vi "Update Indicator Value.vi"(8 "error in (no error)":errorcluster, 9 "uService Template in":refnum<class "Father of all uServices.lvclass">, 10 "Item data":variant, 11 "Control in":refnum<vi>) -> (0 "error out":errorcluster, 3 "Control out":refnum<vi>)   [LabVIEW 2026, in "TALOS.lvlib" / "Father of all uServices.lvlib" / "Father of all uServices.lvclass"]
uses:
  Father of all uServices.lvclass
  Ancestor/Ancestor/Ancestor.lvclass/Ancestor.ctl
  Support VIs/Generate Error.vi
  FGV/Error Memory/Get Error Description.vi
  Support VIs/Get PC name.vi
  Ancestor/Ancestor/Read ID.vi
  Support VIs/Get Class Name.vi
  FGV/Error Memory/Error Memory Core.vi
  <vilib>/AdvancedString/Delimited String to 1D String Array.vi
  <vilib>/AdvancedString/Delimited String to 1D String Array (string).vi
  Support VIs/Circus Root Path.vi
  FGV/Error Memory/Error Crt Lvl checker.vi
  FGV/Error Memory/Error Memory Core.vi/40c8088d-b597-4017-91af-faa98e00292e.vi
  FGV/Error Memory/Error Memory Core.vi/d4a3ab98-063c-4e44-b43d-fbdcfe6c2be2.vi
  Support VIs/Global Memory.vi
  <vilib>/Utility/LVClass/Get LV Class Name.vi
  Support VIs/Is in Packed Library.vi
  Support VIs/TALOS Root path.vi
  Support VIs/Read CSV worksheet.vi
  Support VIs/Global Constants.vi
  <vilib>/Utility/error.llb/General Error Handler.vi
  Support VIs/Error Log.vi
  Ancestor/Ancestor/Ancestor.lvclass
  <vilib>/Comparison/Equal/Equal Functor/Equal Functor.lvclass
  TALOS.lvlib
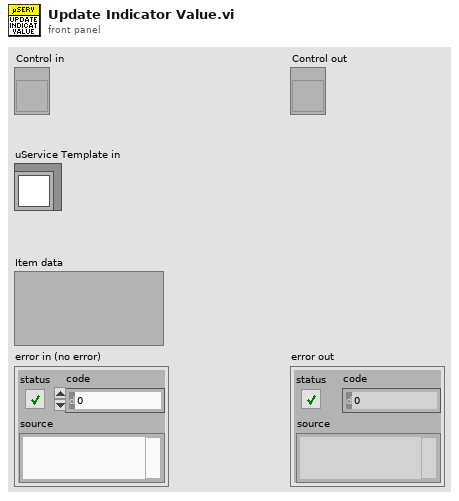
[diagram p1: front panel]
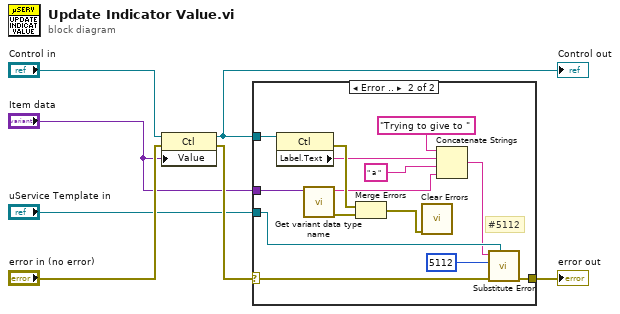
[diagram p0: block diagram]
diagram:
  n1 = property class="Ctl"(reference="Control in", error in="error in (no error)", "Value"="Item data") -> (reference out=w3:refnum<vi>, error out=w5:errorcluster)
  "Control out" <- w3
  n2 = case shown="Error .." w5 {
    selector: w5 -> [w8 w22]
    tunnel: [w8 w21] -> w4
    tunnel: w3 -> [_ w20]
    tunnel: "uService Template in" -> [_ w18]
    tunnel: "Item data" -> [_ w17]
    frame No Error {
    }
    frame Error {
      # "#5112"
      n3 = property class="Ctl"(reference=w20) -> (error out=w16:errorcluster, "Label.Text"=w12:string)  [unwired: 1 in, 1 out]
      n4 = call "Get variant data type name.vi"("variant"=w17) -> ("error out"=w15:errorcluster, "resulting string"=w10:string)  [unwired: 9 in]
      n5 = Merge Errors(w16, w15) -> (w14:errorcluster)
      n6 = call <vilib>:"Clear Errors.vi"("error in (no error)"=w14) -> ()  [unwired: 5 in, 2 out]
      n7 = Concatenate Strings("Trying to give to ", w12, " a ", w10) -> (w9:string)
      n8 = call "Substitute Error.vi"("LabVIEW Object"=w18, "error in (no error)"=w22, "Error Code"=5112, "Optional String"=w9) -> ("error out"=w21:errorcluster)  [unwired: 7 in]
    }
  }
  "error out" <- w4
